vi "Format_Save_2(SubVI).vi"(4 "5 Col":string, 6 "4 Col":string, 7 "1 Col":string, 8 "error in (no error)":errorcluster, 9 "3 Col":string, 10 "2 Col":string, 11 "refnum in":refnum<file>) -> (0 "error out":errorcluster, 3 "refnum out":refnum<file>)   [LabVIEW 2014]
doc: "This SubVI saving data to outter file in same format"
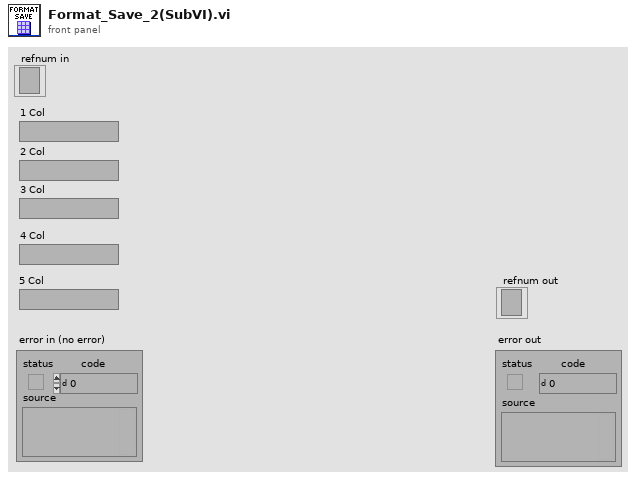
[diagram p1: front panel]
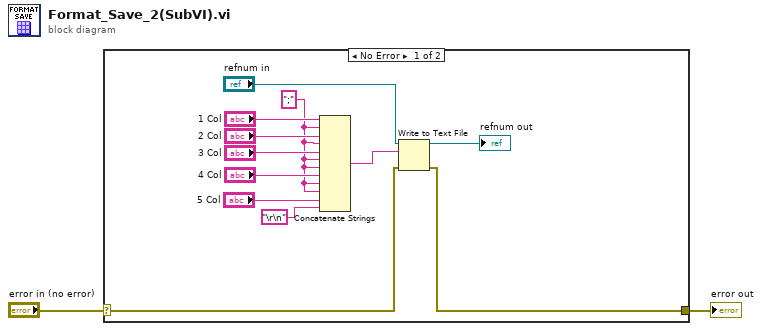
[diagram p0: block diagram]
diagram:
  n1 = case shown="No Error" "error in (no error)" {
    selector: "error in (no error)" -> [w13 w15]
    tunnel: [w12 w15] -> w1
    frame No Error {
      w5 = ";"
      n2 = Concatenate Strings("1 Col", w5, "2 Col", w5, "3 Col", w5, w5, "4 Col", w5, w5, "5 Col", "\r\n") -> (w14:string)
      n3 = Write to Text File(file (use dialog)="refnum in", text=w14, error in=w13) -> (refnum out=→"refnum out":refnum<file>, error out=w12:errorcluster)  [unwired: 1 in, 1 out]
    }
    frame Error {
    }
  }
  "error out" <- w1
